vi "FP Build.vi"(7 "Dry Run?":bool=TRUE, 8 "error in":errorcluster, 11 "Package Version":string="4.57.6.10") -> (0 "Error Out":errorcluster)   [LabVIEW 2019]
uses:
  <vilib>/AppBuilder/AB_API_Simple/Build Specification Version.ctl
  <vilib>/MakerHub/Toolbox/LMH-Toolbox.lvlib
  <vilib>/AppBuilder/AB_API_Simple/NI_App_Builder_API.lvlib
  <userlib>/LevyLab/Build Support/PostBuildSupport/PostBuildSupport.lvclass
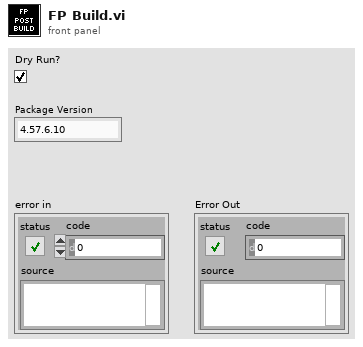
[diagram p1: front panel]
types:
  T1 = typedef "NI_App_Builder_API.lvlib/Build Specification Version.ctl" = cluster{"Major":u16, "Minor":u16, "Fix":u16, "Build":u16}
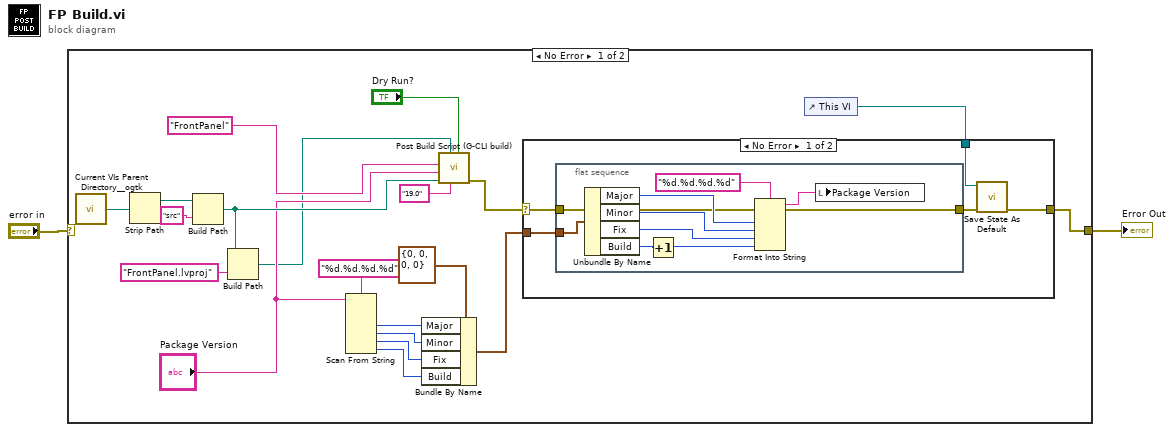
[diagram p0: block diagram]
diagram:
  n1 = case shown="No Error" "error in" {
    selector: "error in" -> [_ w37]
    tunnel: [w10 w37] -> w2
    frame No Error {
      n2 = call <userlib>:"Current VIs Parent Directory__ogtk.vi"() -> ("Parent Directory (+ Relative)"=w22:path)  [unwired: 5 in]
      n3 = Strip Path(path=w22) -> (stripped path=w21:path)  [unwired: 1 out]
      n4 = Build Path(base path=w21, name or relative path="src") -> (appended path=w8:path)
      n5 = Build Path(base path=w8, name or relative path="FrontPanel.lvproj") -> (appended path=w5:path)
      n6 = Scan From String(format string="%d.%d.%d.%d", input string="Package Version") -> (output 1=w14:i32, output 2=w17:i32, output 3=w13:i32, output 4=w16:i32)  [unwired: 6 in, 3 out]
      n7 = Bundle By Name(cluster=T1 {"Major"=0, "Minor"=0, "Fix"=0, "Build"=0} ("Build Specification Version"), "Major"=w14, "Minor"=w17, "Fix"=w13, "Build"=w16) -> (w11:T1)
      n8 = call <userlib>:"Post Build Script (G-CLI build).vi"("create 7zip.bat only [T]"="Dry Run?", "Package LabVIEW Version (19.0 (32-bit))"="19.0", "Project File Path"=w5, "Package Source Folder"=w8, "Package Version (major.minor.patch.build)"="Package Version", "Product Name"="FrontPanel") -> ("error out"=w9:errorcluster)  [unwired: 5 in]
      n9 = control-ref of="This VI"() -> (w19:refnum<vi>)
      n10 = case shown="No Error" w9 {
        selector: w9 -> [w26 _]
        tunnel: w19 -> [w27 _]
        tunnel: w11 -> [w25 _]
        tunnel: [w23 _] -> w10
        frame No Error {
          n11 = flat-sequence {
            tunnel: w26 -> [w28]
            tunnel: w25 -> [w35]
            tunnel: [w28] -> w24
            frame #0 {
              n12 = Unbundle By Name(w35) -> ("Major"=w31:u16, "Minor"=w32:u16, "Fix"=w33:u16, "Build"=w36:u16)
              n13 = Increment(x=w36) -> (x+1=w34:u16)
              n14 = Format Into String(format string="%d.%d.%d.%d", w31, w32, w33, w34) -> (resulting string=w29:string)  [unwired: 2 in, 1 out]
              n15 = local write "Package Version"(w29) -> ()
            }
          }
          n16 = call <vilib>:"Save State As Default.vi"("Error In"=w24, "Target VI"=w27) -> ("Error Out"=w23:errorcluster)  [unwired: 8 in, 1 out]
        }
        frame Error {
        }
      }
    }
    frame Error {
    }
  }
  "Error Out" <- w2
